vi "HFRR ADV v016 new software.vi"() -> ()   [LabVIEW 2025] (continued)
            n3512 = local read "S 49"() -> (w4506:string)
            n3513 = local read "S 52"() -> (w4503:string)
            n3514 = local read "as"() -> (w4488:string)
            n3515 = local read "bs"() -> (w4489:string)
            n3516 = local read "S 56"() -> (w4502:string)
            n3517 = local read "S 57"() -> (w4501:string)
            n3518 = local read "S 58"() -> (w4500:string)
            n3519 = local read "S 59"() -> (w4499:string)
            n3520 = property on="OPEN" class="Bool (strict)"("Boolean Text.Text"=w4503) -> ()  [unwired: 2 in, 2 out]
            n3521 = property on="OPEN 1" class="Bool (strict)"("Boolean Text.Text"=w4507) -> ()  [unwired: 2 in, 2 out]
            n3522 = property on="OPEN 2" class="Bool (strict)"("Boolean Text.Text"=w4506) -> ()  [unwired: 2 in, 2 out]
            n3523 = property on="OPEN 3" class="Bool (strict)"("Boolean Text.Text"=w4505) -> ()  [unwired: 2 in, 2 out]
            n3524 = property on="OPEN 4" class="Bool (strict)"("Boolean Text.Text"=w4504) -> ()  [unwired: 2 in, 2 out]
            n3525 = Concatenate Strings(w4489, "\r", w4488) -> ()  [unwired: 1 out]
            n3526 = local read "S 102"() -> (w4462:string)
            n3527 = property on="КОФ1" class="DigNum (strict)"("Caption.Text"=w4502) -> ()  [unwired: 2 in, 2 out]
            n3528 = local read "S 98"() -> (w4466:string)
            n3529 = local read "S 99"() -> (w4465:string)
            n3530 = local read "S 100"() -> (w4464:string)
            n3531 = local read "S 101"() -> (w4463:string)
            n3532 = property on="КОФ2" class="DigNum (strict)"("Caption.Text"=w4501) -> ()  [unwired: 2 in, 2 out]
            n3533 = property on="КОФ3" class="DigNum (strict)"("Caption.Text"=w4500) -> ()  [unwired: 2 in, 2 out]
            n3534 = property on="КОФ4" class="DigNum (strict)"("Caption.Text"=w4499) -> ()  [unwired: 2 in, 2 out]
            n3535 = local read "bs"() -> (w4487:string)
            n3536 = local read "as"() -> (w4486:string)
            n3537 = property on="CH-POWER +" class="DigNum (strict)"("Caption.Text"=w4466) -> ()  [unwired: 2 in, 2 out]
            n3538 = property on="CH-POWER -" class="DigNum (strict)"("Caption.Text"=w4465) -> ()  [unwired: 2 in, 2 out]
            n3539 = property on="CH-HEATER" class="DigNum (strict)"("Caption.Text"=w4464) -> ()  [unwired: 2 in, 2 out]
            n3540 = property on="CH-HUMIDITY DRY" class="DigNum (strict)"("Caption.Text"=w4463) -> ()  [unwired: 2 in, 2 out]
            n3541 = property on="CH-HUMIDITY WET" class="DigNum (strict)"("Caption.Text"=w4462) -> ()  [unwired: 2 in, 2 out]
            n3542 = local read "S 60"() -> (w4498:string)
            n3543 = local read "S 54"() -> (w4508:string)
            n3544 = Concatenate Strings(w4487, "\r", w4486) -> ()  [unwired: 1 out]
            n3545 = Concatenate Strings(w4508, w4498) -> ()  [unwired: 1 out]
            n3546 = local read "S 77"() -> (→"String 43":string)
            n3547 = local read "S 76"() -> (w4481:string)
            n3548 = local read "S 78"() -> (w4480:string)
            n3549 = local read "S 71"() -> (w4492:string)
            n3550 = local read "S 66"() -> (w4497:string)
            n3551 = local read "S 67"() -> (w4496:string)
            n3552 = local read "S 68"() -> (w4495:string)
            n3553 = local read "S 69"() -> (w4494:string)
            n3554 = local read "S 70"() -> (w4493:string)
            n3555 = property on="AIR TEMP" class="DigNum (strict)"("Caption.Text"=w4480) -> ()  [unwired: 2 in, 2 out]
            n3556 = property on="Set Strk" class="DigNum (strict)"("Caption.Text"=w4481) -> ()  [unwired: 2 in, 2 out]
            n3557 = property on="FRIC. FORCE :" class="DigNum (strict)"("Caption.Text"=w4497) -> ()  [unwired: 2 in, 2 out]
            n3558 = property on="TEMPERATURE :" class="DigNum (strict)"("Caption.Text"=w4496) -> ()  [unwired: 2 in, 2 out]
            n3559 = property on="SPEED OUT:" class="DigNum (strict)"("Caption.Text"=w4495) -> ()  [unwired: 2 in, 2 out]
            n3560 = property on="AIR TEMPERATURE :" class="DigNum (strict)"("Caption.Text"=w4494) -> ()  [unwired: 2 in, 2 out]
            n3561 = property on="HUMIDITY:" class="DigNum (strict)"("Caption.Text"=w4493) -> ()  [unwired: 2 in, 2 out]
            n3562 = property on="EDIT" class="Bool (strict)"("Boolean Text.Text"=w4492) -> ()  [unwired: 2 in, 2 out]
            n3563 = local read "S 79"() -> (w4479:string)
          }
          frame #2 {
          }
        }
        n3564 = local write "Lan flag"(10.0 ("Lan flag")) -> ()
      }
      frame Enabled {
      }
    }
    n3565 = Wait (ms)(milliseconds to wait=u32 2000) -> ()  [unwired: 1 out]
    n3566 = local read "Quit"() -> (w4282:bool)
  }
  n3567 = disable-structure shown="Disabled" {
    frame Disabled {
      n3568 = while {
        tunnel: [w4510] -> _
        i -> [w4510]
        stop <- w4509 continue-if-true
        n3569 = Wait (ms)(milliseconds to wait=u32 50) -> ()  [unwired: 1 out]
        n3570 = stacked-sequence {
          frame #0 {
            # "Controls Text color"
            # "Controls BG color"
            n3571 = property on="FILE" class="Str"("Text.Text Colors:Text Color"="SC  Text") -> ()  [unwired: 2 in, 2 out]
            n3572 = property on="Fuel Discription :" class="Str"("Text.Text Colors:Text Color"="SC  Text") -> ()  [unwired: 2 in, 2 out]
            n3573 = property on="tested by" class="Str"("Text.Text Colors:Text Color"="SC  Text") -> ()  [unwired: 2 in, 2 out]
            n3574 = property on="Remarks :" class="Str"("Text.Text Colors:Text Color"="SC  Text") -> ()  [unwired: 2 in, 2 out]
            n3575 = property class="DigNum (strict)"("Numeric Text.Text Colors:BG Color"="NC BG") -> ()  [unwired: 2 in, 2 out]
            n3576 = property class="DigNum (strict)"("Numeric Text.Text Colors:BG Color"="NC BG") -> ()  [unwired: 2 in, 2 out]
            n3577 = property class="DigNum (strict)"("Numeric Text.Text Colors:BG Color"="NC BG") -> ()  [unwired: 2 in, 2 out]
            n3578 = property class="DigNum (strict)"("Numeric Text.Text Colors:BG Color"="NC BG") -> ()  [unwired: 2 in, 2 out]
            n3579 = property class="DigNum (strict)"("Numeric Text.Text Colors:BG Color"="NC BG") -> ()  [unwired: 2 in, 2 out]
            n3580 = property class="DigNum (strict)"("Numeric Text.Text Colors:BG Color"="NC BG") -> ()  [unwired: 2 in, 2 out]
            n3581 = property class="DigNum (strict)"("Numeric Text.Text Colors:BG Color"="NC BG") -> ()  [unwired: 2 in, 2 out]
            n3582 = property class="DigNum (strict)"("Numeric Text.Text Colors:BG Color"="NC BG") -> ()  [unwired: 2 in, 2 out]
            n3583 = property class="DigNum (strict)"("Numeric Text.Text Colors:BG Color"="NC BG") -> ()  [unwired: 2 in, 2 out]
            n3584 = property class="DigNum (strict)"("Numeric Text.Text Colors:BG Color"="NC BG") -> ()  [unwired: 2 in, 2 out]
            n3585 = property class="DigNum (strict)"("Numeric Text.Text Colors:BG Color"="NC BG") -> ()  [unwired: 2 in, 2 out]
            n3586 = property class="DigNum (strict)"("Numeric Text.Text Colors:BG Color"="NC BG") -> ()  [unwired: 2 in, 2 out]
            n3587 = property on="FILE" class="Str"("Text.Text Colors:BG Color"="SC BG 3") -> ()  [unwired: 2 in, 2 out]
            n3588 = property on="Fuel Discription :" class="Str"("Text.Text Colors:BG Color"="SC BG 3") -> ()  [unwired: 2 in, 2 out]
            n3589 = property on="tested by" class="Str"("Text.Text Colors:BG Color"="SC BG 3") -> ()  [unwired: 2 in, 2 out]
            n3590 = property on="Remarks :" class="Str"("Text.Text Colors:BG Color"="SC BG 3") -> ()  [unwired: 2 in, 2 out]
            n3591 = property class="DigNum (strict)"("Numeric Text.Text Colors:Text Color"="NC Text") -> ()  [unwired: 2 in, 2 out]
            n3592 = property class="DigNum (strict)"("Numeric Text.Text Colors:Text Color"="NC Text") -> ()  [unwired: 2 in, 2 out]
            n3593 = property class="DigNum (strict)"("Numeric Text.Text Colors:Text Color"="NC Text") -> ()  [unwired: 2 in, 2 out]
            n3594 = property class="DigNum (strict)"("Numeric Text.Text Colors:Text Color"="NC Text") -> ()  [unwired: 2 in, 2 out]
            n3595 = property class="DigNum (strict)"("Numeric Text.Text Colors:Text Color"="NC Text") -> ()  [unwired: 2 in, 2 out]
            n3596 = property class="DigNum (strict)"("Numeric Text.Text Colors:Text Color"="NC Text") -> ()  [unwired: 2 in, 2 out]
            n3597 = property class="DigNum (strict)"("Numeric Text.Text Colors:Text Color"="NC Text") -> ()  [unwired: 2 in, 2 out]
            n3598 = property class="DigNum (strict)"("Numeric Text.Text Colors:Text Color"="NC Text") -> ()  [unwired: 2 in, 2 out]
            n3599 = property class="DigNum (strict)"("Numeric Text.Text Colors:Text Color"="NC Text") -> ()  [unwired: 2 in, 2 out]
            n3600 = property class="DigNum (strict)"("Numeric Text.Text Colors:Text Color"="NC Text") -> ()  [unwired: 2 in, 2 out]
            n3601 = property class="DigNum (strict)"("Numeric Text.Text Colors:Text Color"="NC Text") -> ()  [unwired: 2 in, 2 out]
            n3602 = property class="DigNum (strict)"("Numeric Text.Text Colors:Text Color"="NC Text") -> ()  [unwired: 2 in, 2 out]
            n3603 = property class="DigNum (strict)"("Numeric Text.Text Colors:Text Color"="NI Text  2") -> ()  [unwired: 2 in, 2 out]
            n3604 = property class="DigNum (strict)"("Numeric Text.Text Colors:Text Color"="NI Text  2") -> ()  [unwired: 2 in, 2 out]
            n3605 = property class="DigNum (strict)"("Numeric Text.Text Colors:Text Color"="NI Text  2") -> ()  [unwired: 2 in, 2 out]
            n3606 = property class="DigNum (strict)"("Numeric Text.Text Colors:Text Color"="NI Text  2") -> ()  [unwired: 2 in, 2 out]
            n3607 = property class="DigNum (strict)"("Numeric Text.Text Colors:Text Color"="NI Text  2") -> ()  [unwired: 2 in, 2 out]
            n3608 = property class="DigNum (strict)"("Numeric Text.Text Colors:Text Color"="NI Text  2") -> ()  [unwired: 2 in, 2 out]
            n3609 = property class="DigNum (strict)"("Numeric Text.Text Colors:Text Color"="NI Text  2") -> ()  [unwired: 2 in, 2 out]
            n3610 = property class="DigNum (strict)"("Numeric Text.Text Colors:Text Color"="NI Text  2") -> ()  [unwired: 2 in, 2 out]
            n3611 = property class="DigNum (strict)"("Numeric Text.Text Colors:Text Color"="NI Text  2") -> ()  [unwired: 2 in, 2 out]
            n3612 = property class="DigNum (strict)"("Numeric Text.Text Colors:Text Color"="NI Text  2") -> ()  [unwired: 2 in, 2 out]
            n3613 = property class="DigNum (strict)"("Numeric Text.Text Colors:Text Color"="NI Text  2") -> ()  [unwired: 2 in, 2 out]
            n3614 = property class="DigNum (strict)"("Numeric Text.Text Colors:Text Color"="NI Text  2") -> ()  [unwired: 2 in, 2 out]
            n3615 = property class="DigNum (strict)"("Numeric Text.Text Colors:Text Color"="NI Text  2") -> ()  [unwired: 2 in, 2 out]
            n3616 = property class="DigNum (strict)"("Numeric Text.Text Colors:Text Color"="NI Text  2") -> ()  [unwired: 2 in, 2 out]
            n3617 = property class="DigNum (strict)"("Numeric Text.Text Colors:Text Color"="NI Text  2") -> ()  [unwired: 2 in, 2 out]
            n3618 = property on="Coefficient Of Friction" class="XYGraph (strict)"("Plot Area:Colors:FG Color"="GFG  2", "Plot Area:Colors:BG Color"="GBG   2") -> ()  [unwired: 2 in, 2 out]
            n3619 = property on="Humidity ( %RH )" class="XYGraph (strict)"("Plot Area:Colors:FG Color"="GFG  2", "Plot Area:Colors:BG Color"="GBG   2") -> ()  [unwired: 2 in, 2 out]
            n3620 = property on="Air Temperature  ( °C )" class="XYGraph (strict)"("Plot Area:Colors:FG Color"="GFG  2", "Plot Area:Colors:BG Color"="GBG   2") -> ()  [unwired: 2 in, 2 out]
            n3621 = property on="Sample Temperature ( °C )" class="XYGraph (strict)"("Plot Area:Colors:FG Color"="GFG  2", "Plot Area:Colors:BG Color"="GBG   2") -> ()  [unwired: 2 in, 2 out]
            n3622 = property class="DigNum (strict)"("Numeric Text.Text Colors:BG Color"="NI BG 2") -> ()  [unwired: 2 in, 2 out]
            n3623 = property class="DigNum (strict)"("Numeric Text.Text Colors:BG Color"="NI BG 2") -> ()  [unwired: 2 in, 2 out]
            n3624 = property class="DigNum (strict)"("Numeric Text.Text Colors:BG Color"="NI BG 2") -> ()  [unwired: 2 in, 2 out]
            n3625 = property class="DigNum (strict)"("Numeric Text.Text Colors:BG Color"="NI BG 2") -> ()  [unwired: 2 in, 2 out]
            n3626 = property class="DigNum (strict)"("Numeric Text.Text Colors:BG Color"="NI BG 2") -> ()  [unwired: 2 in, 2 out]
            n3627 = property class="DigNum (strict)"("Numeric Text.Text Colors:BG Color"="NI BG 2") -> ()  [unwired: 2 in, 2 out]
            n3628 = property class="DigNum (strict)"("Numeric Text.Text Colors:BG Color"="NI BG 2") -> ()  [unwired: 2 in, 2 out]
            n3629 = property class="DigNum (strict)"("Numeric Text.Text Colors:BG Color"="NI BG 2") -> ()  [unwired: 2 in, 2 out]
            n3630 = property class="DigNum (strict)"("Numeric Text.Text Colors:BG Color"="NI BG 2") -> ()  [unwired: 2 in, 2 out]
            n3631 = property class="DigNum (strict)"("Numeric Text.Text Colors:BG Color"="NI BG 2") -> ()  [unwired: 2 in, 2 out]
            n3632 = property class="DigNum (strict)"("Numeric Text.Text Colors:BG Color"="NI BG 2") -> ()  [unwired: 2 in, 2 out]
            n3633 = property class="DigNum (strict)"("Numeric Text.Text Colors:BG Color"="NI BG 2") -> ()  [unwired: 2 in, 2 out]
            n3634 = property class="DigNum (strict)"("Numeric Text.Text Colors:BG Color"="NI BG 2") -> ()  [unwired: 2 in, 2 out]
            n3635 = property class="DigNum (strict)"("Numeric Text.Text Colors:BG Color"="NI BG 2") -> ()  [unwired: 2 in, 2 out]
            n3636 = property class="DigNum (strict)"("Numeric Text.Text Colors:BG Color"="NI BG 2") -> ()  [unwired: 2 in, 2 out]
            n3637 = property class="Bool"("Colors [4]"="Boolean BC T & BG") -> ()  [unwired: 2 in, 2 out]
            n3638 = property on="Save & Continue" class="Bool (strict)"("Colors [4]"="Boolean BC T & BG") -> ()  [unwired: 2 in, 2 out]
            n3639 = property on="Heater Button" class="Bool (strict)"("Colors [4]"="Boolean BC T & BG") -> ()  [unwired: 2 in, 2 out]
            n3640 = property class="Bool"("Colors [4]"="Boolean BC T & BG") -> ()  [unwired: 2 in, 2 out]
            n3641 = property on="Humidity" class="Bool (strict)"("Colors [4]"="Boolean BC T & BG") -> ()  [unwired: 2 in, 2 out]
            n3642 = property class="Bool (strict)"("Colors [4]"="Boolean BC T & BG") -> ()  [unwired: 2 in, 2 out]
            n3643 = property on="RUN" class="Bool (strict)"("Colors [4]"="Boolean BC T & BG") -> ()  [unwired: 2 in, 2 out]
            n3644 = property on="trip1 8" class="Bool (strict)"("Colors [4]"="Boolean BC T & BG") -> ()  [unwired: 2 in, 2 out]
            n3645 = property class="Bool"("Colors [4]"="Boolean BC T & BG") -> ()  [unwired: 2 in, 2 out]
            n3646 = property class="Bool (strict)"("Colors [4]"="Boolean BC T & BG") -> ()  [unwired: 2 in, 2 out]
            n3647 = property on="OPEN 1" class="Bool (strict)"("Colors [4]"="Boolean BC T & BG 2") -> ()  [unwired: 2 in, 2 out]
            n3648 = property on="OPEN 2" class="Bool (strict)"("Colors [4]"="Boolean BC T & BG 2") -> ()  [unwired: 2 in, 2 out]
            n3649 = property on="OPEN 3" class="Bool (strict)"("Colors [4]"="Boolean BC T & BG 2") -> ()  [unwired: 2 in, 2 out]
            n3650 = property on="OPEN 4" class="Bool (strict)"("Colors [4]"="Boolean BC T & BG 2") -> ()  [unwired: 2 in, 2 out]
            n3651 = property on="OPEN" class="Bool (strict)"("Colors [4]"="Boolean BC T & BG 2") -> ()  [unwired: 2 in, 2 out]
            n3652 = property on="rstv2" class="Bool"("Colors [4]"="Boolean BC T & BG 2") -> ()  [unwired: 2 in, 2 out]
            n3653 = property on="RST CP" class="Bool"("Colors [4]"="Boolean BC T & BG 2") -> ()  [unwired: 2 in, 2 out]
            n3654 = property on="RSTV1 3" class="Bool"("Colors [4]"="Boolean BC T & BG 2") -> ()  [unwired: 2 in, 2 out]
            n3655 = property on="RSTV1 2" class="Bool"("Colors [4]"="Boolean BC T & BG 2") -> ()  [unwired: 2 in, 2 out]
          }
          frame #1 {
          }
        }
        n3656 = local read "Quit"() -> (w4509:bool)
      }
    }
    frame Enabled {
    }
  }
  n3657 = while {
    shift-right: [w4527] -> _
    shift-left: _ -> [w4528]
    shift-right: [w4525] -> _
    shift-left: T19 {"Read Heave and Surge"="", "Bytes at Heave Port"=0.0, "Heave and Surge COM Port:"="COM9", "Com Port 2"="COM7", "Residual Due"="", "Heave COM Status 2"=TRUE, "Heave COM Status"=TRUE, "Port 2"=TRUE, "Sway PPR"=6400.0, "Surge PPR"=6400.0, "Heave PPR"=6400.0, "Sway Pitch"=2.0, "Surge Pitch"=3.0, "Heave Pitch"=4.0, "Sway Pulses/mm"=320.0, "Surge Pulses/mm"=1600.0, "Heave Pulses/mm"=1600.0, "inner loop"=0.0, "Read Heave and Surge 2"="", "String 36"="", "Write S"=FALSE, "WriteCC1"=[""], "Heave COM Loop"=0, "LastCom"="", "EXIT"=FALSE, "Error Heave"={"status"=TRUE, "code"=-1073807343, "source"=""}} -> [w4524]
    shift-right: [w4522] -> _
    shift-left: enum16{"init", "MAIN", "Panel Close"}."init" -> [w4523]
    stop <- w4526 stop-if-true
    n3658 = case shown="\"MAIN\"" w4523 {
      tunnel: w4528 -> [w4542 w4557 w4618 w4620]
      tunnel: [w4536 w4566 w4618 w4620] -> w4527
      tunnel: [_ _ TRUE _] -> w4526
      tunnel: [w4532 w4563 w4616 w4619] -> w4525
      tunnel: w4524 -> [w4539 w4556 w4616 w4619]
      tunnel: [enum16{"init", "MAIN", "Panel Close"}."MAIN" w4550 _ _] -> w4522
      frame "init" {
        n3659 = Bundle By Name(cluster=w4539, "Heave and Surge COM Port:"="C3 :") -> (w4538:T19)
        n3660 = call "Instrument fgv.vi"("Enum"=T31."INIT", "error in (no error) 2"=w4542, "INPUT"=w4538) -> ("error"=w4540:errorcluster, "output"=w4535:T19)  [unwired: 6 in, 1 out]
        n3661 = case shown="Error" w4540 {
          selector: w4540 -> [w4544 _]
          tunnel: [w4544 w4548] -> w4536
          tunnel: w4535 -> [w4543 w4546]
          tunnel: [w4543 w4545] -> w4533
          frame No Error {
          }
          frame Error {
            n3662 = call "Instrument fgv.vi"("Enum"=T31."ERROR INIT", "INPUT"=w4546) -> ("error"=w4549:errorcluster, "output"=w4545:T19)  [unwired: 7 in, 1 out]
            n3663 = call <vilib>:"Clear Errors.vi"("error in (no error)"=w4549) -> ("error out"=w4548:errorcluster)  [unwired: 5 in, 1 out]
          }
        }
        n3664 = local read "LastCom"() -> (w4531:string)
        n3665 = Unbundle By Name(w4533) -> ("Heave COM Status 2"=→"COM Status" →"Instrument Status":bool, "Error Heave"=→"Error":errorcluster)  [unwired: 1 out]
        n3666 = Bundle By Name(cluster=w4533, "LastCom"=w4531) -> (w4532:T19)
      }
      frame "MAIN" {
        n3667 = Unbundle By Name(w4556) -> ("Com Port 2"=w4568:refnum<visa-resource-name>)
        n3668 = local write "Com Port 4"(w4568) -> ()
        n3669 = local read "C3 :"() -> (w4554:refnum<visa-resource-name>)
        n3670 = Bundle By Name(cluster=w4556, "Heave and Surge COM Port:"=w4554) -> (w4555:T19)
        n3671 = Equal?(x=w4568, y=w4554) -> (x = y?=w4567:bool)
        n3672 = case shown="True" w4567 {
          tunnel: [w4572 w4589] -> w4566
          tunnel: w4557 -> [w4573 w4595]
          tunnel: w4555 -> [w4571 w4593]
          tunnel: [w4570 w4588] -> w4563
          frame False {
            n3673 = call <vilib>:"Clear Errors.vi"("error in (no error)"=w4573) -> ("error out"=w4569:errorcluster)  [unwired: 5 in, 1 out]
            n3674 = call "Instrument fgv.vi"("Enum"=T31."ERROR INIT", "error in (no error) 2"=w4569, "INPUT"=w4571) -> ("error"=w4575:errorcluster, "output"=w4570:T19)  [unwired: 6 in, 1 out]
            n3675 = call <vilib>:"Clear Errors.vi"("error in (no error)"=w4575) -> ("error out"=w4572:errorcluster)  [unwired: 5 in, 1 out]
          }
          frame True {
            n3676 = call "Instrument fgv.vi"("Enum"=T31."READ", "error in (no error) 2"=w4595, "INPUT"=w4593) -> ("error"=w4594:errorcluster, "output"=w4585:T19)  [unwired: 6 in, 1 out]
            n3677 = Bundle By Name(cluster=w4585, "String 36"="String 11") -> (w4584:T19)
            n3678 = case shown="True" "Write S" {
              selector: "Write S" -> [_ w4615]
              tunnel: w4594 -> [w4608 w4614]
              tunnel: [w4608 w4613] -> w4581
              tunnel: w4584 -> [w4607 w4610]
              tunnel: [w4607 w4609] -> w4580
              frame False {
              }
              frame True {
                n3679 = Not(x=w4615) -> (.not. x?=w4611:bool)
                n3680 = local write "Write S"(w4611) -> ()
                n3681 = call "Instrument fgv.vi"("Enum"=T31."MANUAL WRITE", "error in (no error) 2"=w4614, "INPUT"=w4610) -> ("error"=w4613:errorcluster, "output"=w4609:T19)  [unwired: 6 in, 1 out]
              }
            }
            n3682 = Array Size(array="WriteHumidity") -> (size(s)=w4578:i32)
            n3683 = Greater Than 0?(x=w4578) -> (x > 0?=w4576:bool)
            n3684 = call "Instrument fgv.vi"("Enum"=T31."WRITE", "error in (no error) 2"=w4581, "WriteCC1"="WriteHumidity", "INPUT"=w4580) -> ("error"=w4591:errorcluster, "WriteCC1 2"=w4579:string[], "output"=w4590:T19)  [unwired: 5 in]
            n3685 = case shown="True" w4576 {
              tunnel: w4579 -> [_ w4597]
              frame False {
              }
              frame True {
                n3686 = local write "WriteHumidity"(w4597) -> ()
              }
            }
            n3687 = case shown="Error" w4591 {
              selector: w4591 -> [w4598 w4601]
              tunnel: w4590 -> [w4599 w4606]
              tunnel: [w4599 w4605] -> w4588
              tunnel: [w4598 w4603] -> w4589
              frame No Error {
              }
              frame Error {
                n3688 = call <vilib>:"Clear Errors.vi"("error in (no error)"=w4601) -> ("error out"=w4600:errorcluster)  [unwired: 5 in, 1 out]
                n3689 = call "Instrument fgv.vi"("Enum"=T31."ERROR INIT", "error in (no error) 2"=w4600, "INPUT"=w4606) -> ("error"=w4604:errorcluster, "output"=w4605:T19)  [unwired: 6 in, 1 out]
                n3690 = call <vilib>:"Clear Errors.vi"("error in (no error)"=w4604) -> ("error out"=w4603:errorcluster)  [unwired: 5 in, 1 out]
              }
            }
            n3691 = Unbundle By Name(w4588) -> ("LastCom"=→"LastCom":string, "Read Heave and Surge"=→"Read Humidity":string)
          }
        }
        n3692 = Unbundle By Name(w4563) -> ("Heave COM Status 2"=w4565:bool, "Heave COM Status"=w4564:bool, "Error Heave"=w4561:errorcluster, "Bytes at Heave Port"=→"Bytes at Humidity Port":dbl)
        n3693 = Unbundle By Name(w4561) -> ("status"=→"Humidity Port":bool)
        n3694 = Not(x=w4564) -> (.not. x?=w4558:bool)
        n3695 = local write "Error"(w4561) -> ()
        n3696 = Not(x=w4565) -> (.not. x?=w4559:bool)
        n3697 = local write "Instrument Status"(w4558) -> ()
        n3698 = local write "COM Status"(w4559) -> ()
        n3699 = local read "Quit"() -> (w4551:bool)
        n3700 = Select(t=enum16{"init", "MAIN", "Panel Close"}."Panel Close", s=w4551, f=enum16{"init", "MAIN", "Panel Close"}."MAIN") -> (s? t:f=w4550:enum16{"init", "MAIN", "Panel Close"})
      }
      frame "Panel Close" {
      }
      frame Default {
      }
    }
  }
  n3701 = while {
    stop <- w4646 stop-if-true
    n3702 = local read "Read Humidity"() -> (w4627:string)
    n3703 = call <vilib>:"High Resolution Polling Wait.vi"("seconds to wait"=0.1) -> ()  [unwired: 10 in, 1 out]
    n3704 = Spreadsheet String To Array(delimiter (Tab)=",", format string="", spreadsheet string=w4627, array type (2D Dbl)=string[] []) -> (array=w4641:string[])
    n3705 = for {
      tunnel: w4641 -> [w4651] mode=indexing
      tunnel: string[] ["STATE;", "SET;", "RH;", "T;", "AMB_RH;", "AMB_T;", "PUMP;", "FAN_IN;", "FAN_OUT;", "DEHUM;", "CURRENT;", "STALL;"] -> [w4650] mode=indexing
      tunnel: [w4649] -> w4640 mode=indexing
      n3706 = Match Pattern(string=w4651, regular expression=w4650) -> (after substring=w4649:string)  [unwired: 1 in, 3 out]
    }
    n3707 = Index Array(array=w4640) -> (element #1=→"STATE :":string, element #2=→"SET :":string, element #3=w4629:string, element #4=→"T :":string, element #5=w4626:string, element #6=→"AMB_T :":string, element #7=→"PUMP :":string, element #8=→"FAN_IN :":string, element #9=→"FAN_OUT :":string, element #10=→"DEHUM :":string, element #11=→"CURRENT :":string, element #12=→"STALL :":string)  [unwired: 12 in]
    "RH :" <- w4629
    "AMB_RH :" <- w4626
    n3708 = Fract/Exp String To Number(string=w4629) -> (number=w4621:dbl)  [unwired: 3 in, 1 out]
    n3709 = Fract/Exp String To Number(string=w4626) -> (number=w4625:dbl)  [unwired: 3 in, 1 out]
    n3710 = local write "Ambient Humidity :"(w4625) -> ()
    n3711 = Equal?(x=w4621, y=0.0) -> (x = y?=w4623:bool)
    n3712 = case shown="True" w4623 {
      tunnel: [w4647 w4648] -> w4622
      tunnel: w4621 -> [w4647 _]
      frame False {
        (unwired) 0.0
        "Humidity temp" <- w4647
      }
      frame True {
        n3713 = local read "Humidity temp"() -> (w4648:dbl)
      }
    }
    "RH Numeric:" <- w4622
    n3714 = local read "Quit"() -> (w4646:bool)
  }
  n3715 = disable-structure shown="Disabled" {
    frame Disabled {
      n3716 = while {
        tunnel: [w4885] -> _
        i -> [w4885]
        stop <- w4882 stop-if-true
        n3717 = local read "powstat"() -> (w4883:bool)
        n3718 = case shown="True" w4883 {
          frame False {
          }
          frame True {
            n3719 = local read "RUN"() -> (w4886:bool)
            n3720 = case shown="True" w4886 {
              frame False {
                w4916 = 65.0 ("y")
                n3721 = local read "Set Hz"() -> (w4944:dbl)
                n3722 = local read "NORMAL LOAD"() -> (w4945:dbl)
                n3723 = Multiply(x=w4944, y=60.0) -> (x*y=w4951:dbl)
                n3724 = Multiply(x=1.2 ("y"), y=0.949) -> (x*y=w4920:dbl)
                n3725 = Multiply(x=1.2 ("y"), y=0.8166) -> (x*y=w4924:dbl)
                n3726 = Multiply(x=1.2 ("y"), y=0.851) -> (x*y=w4919:dbl)
                n3727 = local read "FF 2"() -> (w4943:dbl)
                n3728 = Absolute Value(x=w4951) -> (abs(x)=w4949:dbl)
                n3729 = case shown="13.." w4943 {
                  tunnel: [1 2 3] -> w4941
                  frame 0..10, Default {
                    # "Normal"
                  }
                  frame 11, 12 {
                  }
                  frame 13.. {
                  }
                }
                "FF STATE" <- w4941
                n3730 = local read "TEMP"() -> (w4904:dbl)
                n3731 = local read item#-1() -> (w4918)
                n3732 = Less?(x=w4918, y=w4924) -> (x < y?=w4921:bool)
                n3733 = In Range and Coerce(upper limit=w4920, x=w4918, lower limit=w4919) -> (In Range?=w4922:bool)  [unwired: 1 out]
                n3734 = case shown="3601.." w4949 {
                  tunnel: [1 2 3] -> w4947
                  frame 0..3000, Default {
                    # "Normal"
                  }
                  frame 3001..3600 {
                  }
                  frame 3601.. {
                  }
                }
                n3735 = case shown="11.." w4945 {
                  tunnel: [1 3] -> w4946
                  frame 1..10, Default {
                  }
                  frame 11.. {
                  }
                }
                "NL STATE" <- w4946
                n3736 = Multiply(x=1.2 ("y"), y=0.95) -> (x*y=w4934:dbl)
                n3737 = Multiply(x=w4916, y=0.954) -> (x*y=w4908:dbl)
                n3738 = Or(x=w4921, y=w4922) -> (x .or. y?=w4923:bool)
                n3739 = Greater Or Equal?(x=w4918, y=w4934) -> (x >= y?=w4931:bool)
                n3740 = Multiply(x=w4916, y=0.99) -> (x*y=w4905:dbl)
                n3741 = Greater Or Equal?(x=w4904, y=w4905) -> (x >= y?=w4910:bool)
                n3742 = Greater Or Equal?(x=w4904, y=w4908) -> (x >= y?=w4907:bool)
                n3743 = case shown="0, 1, Default" w4918 {
                  tunnel: [1 3] -> w4935
                  frame 0, 1, Default {
                  }
                  frame 2.. {
                  }
                }
                n3744 = case shown="True" w4931 {
                  tunnel: [1 3] -> w4936
                  frame False {
                  }
                  frame True {
                  }
                }
                n3745 = case shown="True" w4923 {
                  tunnel: [1 2] -> w4937
                  frame False {
                  }
                  frame True {
                  }
                }
                n3746 = case shown="..0" w4904 {
                  tunnel: [2 3 3 1] -> w4911
                  frame 61, 62 {
                  }
                  frame 63.. {
                  }
                  frame ..0 {
                  }
                  frame 10..60, Default {
                  }
                }
                n3747 = case shown="True" w4910 {
                  tunnel: [1 3] -> w4912
                  frame False {
                  }
                  frame True {
                  }
                }
                n3748 = Number To Decimal String(number=w4947) -> (decimal integer string=w4948:string)  [unwired: 1 in]
                n3749 = case shown="True" w4907 {
                  tunnel: [1 2] -> w4913
                  frame False {
                  }
                  frame True {
                  }
                }
                n3750 = Number To Decimal String(number=1) -> (decimal integer string=→"Air temp":string)  [unwired: 1 in]
                n3751 = Number To Decimal String(number=w4941) -> (decimal integer string=→"ff_st":string)  [unwired: 1 in]
                n3752 = local write "sp_st"(w4948) -> ()
                n3753 = Number To Decimal String(number=w4946) -> (decimal integer string=→"nl_st":string)  [unwired: 1 in]
                n3754 = Build Array(w4911, w4912, w4913) -> (w4914:i32[])
                n3755 = Build Array(w4935, w4936, w4937) -> (w4938:i32[])
                n3756 = Array Max & Min(array=w4914) -> (max value=w4915:i32)  [unwired: 3 out]
                n3757 = Array Max & Min(array=w4938) -> (max value=w4939:i32)  [unwired: 3 out]
                n3758 = Number To Decimal String(number=w4915) -> (decimal integer string=w4903:string)  [unwired: 1 in]
                n3759 = Number To Decimal String(number=w4939) -> (decimal integer string=→"Stroke Ln 2":string)  [unwired: 1 in]
                n3760 = local write "temp_st"(w4903) -> ()
              }
              frame True {
                w5001 = 65.0 ("y")
                # "Healthy -1\nWarning -2\nError -3"
                n3761 = local read "TEMP"() -> (w5012:dbl)
                n3762 = local read "NORMAL LOAD"() -> (w5016:dbl)
                n3763 = local read "Set Hz"() -> (w5014:dbl)
                n3764 = Multiply(x=1.2 ("y"), y=0.949) -> (x*y=w4996:dbl)
                n3765 = Multiply(x=1.2 ("y"), y=0.8166) -> (x*y=w4992:dbl)
                n3766 = Multiply(x=1.2 ("y"), y=0.851) -> (x*y=w4997:dbl)
                n3767 = Multiply(x=w5001, y=0.954) -> (x*y=w5008:dbl)
                n3768 = Multiply(x=w5001, y=0.99) -> (x*y=w5011:dbl)
                n3769 = Greater Or Equal?(x=w5012, y=w5011) -> (x >= y?=w5006:bool)
                n3770 = Multiply(x=w5014, y=60.0) -> (x*y=w5020:dbl)
                n3771 = Greater Or Equal?(x=w5012, y=w5008) -> (x >= y?=w5009:bool)
                n3772 = local read "FF 2"() -> (w5015:dbl)
                n3773 = local read item#-1() -> (w4998)
                n3774 = Less?(x=w4998, y=w4992) -> (x < y?=w4995:bool)
                n3775 = In Range and Coerce(upper limit=w4996, x=w4998, lower limit=w4997) -> (In Range?=w4994:bool)  [unwired: 1 out]
                n3776 = Absolute Value(x=w5020) -> (abs(x)=w5018:dbl)
                n3777 = case shown="63.." w5012 {
                  tunnel: [2 3 3 1] -> w5005
                  frame 61, 62 {
                  }
                  frame 63.. {
                  }
                  frame ..0 {
                  }
                  frame 10..60, Default {
                  }
                }
                n3778 = case shown="True" w5006 {
                  tunnel: [1 3] -> w5004
                  frame False {
                  }
                  frame True {
                  }
                }
                n3779 = case shown="True" w5009 {
                  tunnel: [1 2] -> w5003
                  frame False {
                  }
                  frame True {
                  }
                }
                n3780 = Multiply(x=1.2 ("y"), y=0.95) -> (x*y=w4982:dbl)
                n3781 = case shown="1..10, Default" w5016 {
                  tunnel: [1 3] -> w5023
                  frame 1..10, Default {
                  }
                  frame 11.. {
                  }
                }
                n3782 = case shown="0..10, Default" w5015 {
                  tunnel: [1 2 3] -> w5022
                  frame 0..10, Default {
                  }
                  frame 11, 12 {
                  }
                  frame 13.. {
                  }
                }
                n3783 = case shown="3601.." w5018 {
                  tunnel: [1 2 3] -> w5017
                  frame 0..3000, Default {
                    # "Normal"
                  }
                  frame 3001..3600 {
                  }
                  frame 3601.. {
                  }
                }
                n3784 = Or(x=w4995, y=w4994) -> (x .or. y?=w4993:bool)
                n3785 = Greater Or Equal?(x=w4998, y=w4982) -> (x >= y?=w4985:bool)
                n3786 = case shown="0, 1, Default" w4998 {
                  tunnel: [1 3] -> w4981
                  frame 0, 1, Default {
                  }
                  frame 2.. {
                  }
                }
                n3787 = case shown="True" w4985 {
                  tunnel: [1 3] -> w4980
                  frame False {
                  }
                  frame True {
                  }
                }
                n3788 = case shown="True" w4993 {
                  tunnel: [1 2] -> w4979
                  frame False {
                  }
                  frame True {
                  }
                }
                n3789 = Build Array(w5005, w5004, w5003) -> (w5002:i32[])
                n3790 = Number To Decimal String(number=w5017) -> (decimal integer string=→"sp_st":string)  [unwired: 1 in]
                n3791 = Array Max & Min(array=w5002) -> (max value=w4999:i32)  [unwired: 3 out]
                "TEMP STATE" <- w4999
                n3792 = Number To Decimal String(number=w5023) -> (decimal integer string=w5026:string)  [unwired: 1 in]
                n3793 = Number To Decimal String(number=w5022) -> (decimal integer string=w5024:string)  [unwired: 1 in]
                n3794 = Number To Decimal String(number=w4999) -> (decimal integer string=→"temp_st":string)  [unwired: 1 in]
                n3795 = Build Array(w4981, w4980, w4979) -> (w4978:i32[])
                n3796 = local write "nl_st"(w5026) -> ()
                n3797 = local write "ff_st"(w5024) -> ()
                n3798 = Number To Decimal String(number=1) -> (decimal integer string=w5021:string)  [unwired: 1 in]
                n3799 = Array Max & Min(array=w4978) -> (max value=w4977:i32)  [unwired: 3 out]
                n3800 = local write "Air temp"(w5021) -> ()
                n3801 = Number To Decimal String(number=w4977) -> (decimal integer string=w4976:string)  [unwired: 1 in]
                n3802 = local write "Stroke Ln 2"(w4976) -> ()
              }
            }
            n3803 = local read "Stroke Ln 2"() -> (w4888:string)
            n3804 = local read "nl_st"() -> (w4894:string)
            n3805 = local read "ff_st"() -> (w4891:string)
            n3806 = local read "sp_st"() -> (w4892:string)
            n3807 = local read "temp_st"() -> (w4893:string)
            n3808 = local read "Air temp"() -> (w4887:string)
            n3809 = Replace Array Subset(array="in", new element #1=w4894, index #1=1 ("index"), new element #2=w4891, index #2=2 ("index"), new element #3=w4893, index #3=3 ("index"), new element #4=w4892, index #4=4 ("index"), new element #5=w4888, index #5=5 ("index"), new element #6=w4887, index #6=6 ("index"), new element #7="Sensor State" ("new element/subarray"), index #7=0 ("index")) -> (→"out":string[])
          }
        }
        n3810 = Wait (ms)(milliseconds to wait=u32 10) -> ()  [unwired: 1 out]
        n3811 = local read "Quit"() -> (w4882:bool)
      }
      n3812 = while {
        stop <- w4857 stop-if-true
        n3813 = local read "run replace"() -> (w4859:bool)
        n3814 = Wait (ms)(milliseconds to wait=u32 100) -> ()  [unwired: 1 out]
        n3815 = Equal?(x="FLAG 2", y=0.0) -> (x = y?=w4860:bool)
        n3816 = case shown="True" w4860 {
          frame False {
          }
          frame True {
            n3817 = local write "FLAG 2"(100.0 ("FLAG 2")) -> ()
            n3818 = call <vilib>:"Read Characters From File.vi"("file path (dialog if empty)"=path "C:/LAB-IQ-NXT/WO 2449 TT.sig", "convert eol? (no:F)"=FALSE ("append to file? (new file:F)")) -> ("character string"=w4863:string)  [unwired: 4 in, 3 out]
            n3819 = call <vilib>:"Read Characters From File.vi"("file path (dialog if empty)"=path "C:/LAB-IQ-NXT/WO 2449 TRH.sig", "convert eol? (no:F)"=FALSE ("append to file? (new file:F)")) -> ("character string"=w4864:string)  [unwired: 4 in, 3 out]
            n3820 = Decimal String To Number(string=w4863) -> (number=w4865:i32)  [unwired: 2 in, 1 out]
            n3821 = local write "Total No. of Tests"(w4865) -> ()
            n3822 = Decimal String To Number(string=w4864) -> (number=w4868:i32)  [unwired: 2 in, 1 out]
            n3823 = local write "SEN.RUN HRS"(w4868) -> ()
          }
        }
        n3824 = case shown="True" w4859 {
          frame False {
          }
          frame True {
            n3825 = Equal?(x="FLAG 4", y=0.0) -> (x = y?=w4872:bool)
            n3826 = case shown="False" w4872 {
              frame False {
                n3827 = Get Date/Time In Seconds() -> (seconds since 1Jan1904=w4878:timestamp)
                n3828 = local read "START 3"() -> (w4876:dbl)
                n3829 = To Double Precision Float(number=w4878) -> (double precision float=w4877:dbl)
                n3830 = Subtract(x=w4877, y=w4876) -> (x-y=→"SENSOR TIME":dbl)
              }
              frame True {
                n3831 = Get Date/Time In Seconds() -> (seconds since 1Jan1904=w4880:timestamp)
                n3832 = local write "FLAG 4"(100.0 ("FLAG")) -> ()
                n3833 = To Double Precision Float(number=w4880) -> (double precision float=→"START 3":dbl)
              }
            }
          }
        }
        n3834 = local read "Quit"() -> (w4857:bool)
      }
      n3835 = while {
        shift-right: [w4657] -> _
        shift-left: _ -> [w4658]
        tunnel: [w4653] -> _
        i -> [w4653]
        stop <- w4652 stop-if-true
        n3836 = Wait (ms)(milliseconds to wait=u32 50 ("Refresh Rate (ms)")) -> ()  [unwired: 1 out]
        n3837 = local read "Json End Flg"() -> (w4654:bool)
        n3838 = Not(x="Upld AR 2") -> ()  [unwired: 1 out]
        n3839 = local read "Upld AR 2"() -> (w4655:bool)
        n3840 = call "Elapsed Time9"("Time Target (s)"="Sen.Upload Rate (s)", "Reset"=FALSE, "Auto Reset"=TRUE) -> ("Time has Elapsed"=w4664:bool)  [unwired: 9 in, 7 out]
        n3841 = Or(x=w4664, y=w4654) -> (x .or. y?=w4660:bool)
        n3842 = case shown="True" w4660 {
          frame False {
          }
          frame True {
            w4756 = "\"SensorName\":\"" ("string")
            w4726 = " \"},{"
            w4751 = "\",\"SensorState\":\""
            w4753 = "\",\"SensorModelNumber\":\"" ("string")
            w4752 = "\",\"SensorRuntimeHours\":\"" ("string")
            n3843 = local read "model num"() -> (w4750:string[])
            n3844 = local read "Sensor name"() -> (w4769:string[])
            n3845 = local read "run"() -> (w4740:string[])
            n3846 = local read "SENSOR TIME"() -> (w4696:dbl)
            n3847 = local read "out"() -> (w4689:string[])
            n3848 = local read "Total No. of Tests"() -> (w4694:dbl)
            n3849 = Select(t=60.0, s="Run test 3", f=3600.0) -> (s? t:f=w4704:dbl)
            n3850 = Index Array(array=w4750, index #1=1 ("index")) -> (element #1=w4749:string, element #2=w4748:string, element #3=w4747:string, element #4=w4746:string, element #5=w4745:string, element #6=w4744:string)  [unwired: 5 in]
            n3851 = Index Array(array=w4740, index #1=1 ("index")) -> (element #1=w4739:string, element #2=w4738:string, element #3=w4737:string, element #4=w4736:string, element #5=w4735:string, element #6=w4734:string)  [unwired: 5 in]
            n3852 = Index Array(array=w4769, index #1=1 ("index")) -> (element #1=w4768:string, element #2=w4767:string, element #3=w4766:string, element #4=w4765:string, element #5=w4755:string, element #6=w4754:string)  [unwired: 5 in]
            n3853 = Index Array(array=w4689, index #1=1 ("index")) -> (element #1=w4721:string, element #2=w4720:string, element #3=w4719:string, element #4=w4718:string, element #5=w4717:string, element #6=w4716:string)  [unwired: 5 in]
            n3854 = local read "SEN.RUN HRS"() -> (w4692:dbl)
            n3855 = Divide(x=w4696, y=w4704) -> (x/y=w4703:dbl)
            n3856 = Increment(x=w4703) -> (x+1=w4699:dbl)
            n3857 = Number To Decimal String(number=w4699) -> (decimal integer string=→"run hrs":string)  [unwired: 1 in]
            n3858 = Divide(x=w4692, y=3600.0 ("f")) -> (x/y=w4687:dbl)
            n3859 = Round To Nearest(number=w4687) -> (nearest integer value=w4685:dbl)
            n3860 = Number To Decimal String(number=w4685) -> (decimal integer string=w4686:string)  [unwired: 1 in]
            n3861 = Number To Decimal String(number=w4694) -> (decimal integer string=w4695:string)  [unwired: 1 in]
            n3862 = local read "Model No"() -> (w4700:string)
            n3863 = local read "UUID"() -> (w4795:string)
            n3864 = local read "Serial No"() -> (w4799:string)
            n3865 = local read "Secret Key"() -> (w4800:string)
            n3866 = Concatenate Strings("\",\"MachineSerialNumber\":\"" ("string"), w4799) -> (w4803:string)
            n3867 = Concatenate Strings("\",\"ModelNumber\":\"" ("string"), w4700) -> (w4701:string)
            n3868 = Concatenate Strings("\",\"MachineRuntimeHours\":\"" ("string"), w4686) -> (w4804:string)
            n3869 = Concatenate Strings("\",\"MachineRuntimeCycles\":\"", w4695) -> (w4797:string)
            n3870 = Concatenate Strings(w4753, w4749) -> (w4783:string)
            n3871 = Concatenate Strings(w4752, w4739) -> (w4784:string)
            n3872 = Concatenate Strings(w4751, w4721) -> (w4782:string)
            n3873 = Concatenate Strings(w4803, w4701, w4804, w4797) -> (w4806:string)
            n3874 = Concatenate Strings(w4753, w4748) -> (w4780:string)
            n3875 = Concatenate Strings(w4752, w4738) -> (w4779:string)
            n3876 = Concatenate Strings(w4751, w4720) -> (w4781:string)
            n3877 = Concatenate Strings(w4753, w4747) -> (w4775:string)
            n3878 = Concatenate Strings(w4752, w4737) -> (w4776:string)
            n3879 = Concatenate Strings(w4751, w4719) -> (w4774:string)
            n3880 = Concatenate Strings(w4753, w4746) -> (w4772:string)
            n3881 = Concatenate Strings(w4752, w4736) -> (w4771:string)
            n3882 = Concatenate Strings(w4751, w4718) -> (w4773:string)
            n3883 = Concatenate Strings(w4783, w4784, w4782) -> (w4785:string)
            n3884 = Concatenate Strings(w4753, w4745) -> (w4762:string)
            n3885 = Concatenate Strings(w4752, w4735) -> (w4763:string)
            n3886 = Concatenate Strings(w4753, w4744) -> (w4759:string)
            n3887 = Concatenate Strings(w4752, w4734) -> (w4758:string)
            n3888 = Concatenate Strings(w4751, w4717) -> (w4761:string)
            n3889 = Concatenate Strings(w4751, w4716) -> (w4760:string)
            n3890 = Concatenate Strings("{\"SecretKey\":\"", w4800, w4806, "\",\"UUID\" : \"", w4795, "\",\"SensorInformation\":", "[{" ("string")) -> (w4733:string)
            n3891 = Concatenate Strings(w4780, w4779, w4781) -> (w4778:string)
            n3892 = Concatenate Strings(w4775, w4776, w4774) -> (w4777:string)
            n3893 = Concatenate Strings(w4772, w4771, w4773) -> (w4770:string)
            n3894 = Concatenate Strings(w4762, w4763, w4761) -> (w4764:string)
            n3895 = Concatenate Strings(w4759, w4758, w4760) -> (w4757:string)
            n3896 = Concatenate Strings(w4756, w4768, w4785, w4726) -> (w4732:string)
            n3897 = Concatenate Strings(w4756, w4767, w4778, w4726) -> (w4731:string)
            n3898 = Concatenate Strings(w4756, w4766, w4777, w4726) -> (w4730:string)
            n3899 = Concatenate Strings(w4756, w4765, w4770, w4726) -> (w4729:string)
            n3900 = Concatenate Strings(w4756, w4755, w4764, w4726) -> (w4728:string)
            n3901 = Concatenate Strings(w4756, w4754, w4757, "\"}" ("string")) -> (w4727:string)
            n3902 = Concatenate Strings(w4733, w4732, w4731, w4730, w4729, w4728, w4727, "]}" ("string")) -> (w4724:string)
            n3903 = local read "SEN.RUN HRS"() -> (w4691:dbl)
            n3904 = disable-structure shown="Disabled" {
              frame Disabled {
                n3905 = local read "state"() -> (w4810:string[])
                n3906 = Delete From Array(array=w4810, index=0) -> (array with subset deleted=w4808:string[])  [unwired: 1 in, 1 out]
                n3907 = for {
                  N: 6 -> [_]
                  tunnel: w4808 -> [w4821] mode=indexing
                  tunnel: [w4820] -> w4807 mode=indexing
                  n3908 = Equal?(x=w4821, y="Warning") -> (x = y?=w4817:bool)
                  n3909 = Equal?(x=w4821, y="Healthy") -> (x = y?=w4814:bool)
                  n3910 = Select(t="2" ("y"), s=w4817, f="3" ("y")) -> (s? t:f=w4812:string)
                  n3911 = Select(t="1" ("y"), s=w4814, f=w4812) -> (s? t:f=w4820:string)
                }
                "state1" <- w4807
              }
              frame Enabled {
              }
            }
            n3912 = stacked-sequence {
              tunnel: w4724 -> [w4832 _ _]
              tunnel: [_ _ w4848] -> _
              frame #0 {
                (unwired) FALSE ("convert eol (F)")
                w4834 = enum16{"start", "end", "current"}."start" ("pos mode (0:2)")
                n3913 = local read "Path"() -> (w4828:path)
                n3914 = Path To String(path=w4828) -> (string=w4840:string)
                n3915 = Concatenate Strings(w4840, "\\", "Sensor File Name") -> (w4841:string)
                n3916 = local write "standard output 2"(" ") -> ()
                n3917 = String To Path(string=w4841) -> (path=w4831:path)
                n3918 = call <vilib>:"Open_Create_Replace File.vi"("advisory dialog? (display:T)"=FALSE, "function (open:0)"=T32."create or replace", "file path"=w4831) -> ("error out"=w4844:errorcluster, "refnum"=w4843:refnum<file>)  [unwired: 5 in, 2 out]
                n3919 = Set File Position(refnum=w4843, from (0:start)=w4834, error in=w4844) -> (refnum out=w4824:refnum<file>, error out=w4823:errorcluster)  [unwired: 1 in]
                n3920 = Write to Binary File(file (use dialog)=w4824, data=" ", error in=w4823, 5:FALSE ("prepend array or string size? (T)")) -> (refnum out=w4835:refnum<file>, error out=w4836:errorcluster)  [unwired: 2 in, 1 out]
                n3921 = Set File Position(offset (in bytes) (0)=w4834, refnum=w4835, error in=w4836) -> (refnum out=w4827:refnum<file>, error out=w4826:errorcluster)  [unwired: 1 in]
                n3922 = Write to Binary File(file (use dialog)=w4827, data=w4832, error in=w4826, 5:FALSE ("prepend array or string size? (T)")) -> (error out=w4830:errorcluster)  [unwired: 2 in, 2 out]
                n3923 = flat-sequence {
                  tunnel: w4831 -> [w4846]
                  tunnel: w4830 -> [_]
                  frame #0 {
                    n3924 = call <vilib>:"Read Characters From File.vi"("file path (dialog if empty)"=w4846) -> ("character string"=→"Sensor Health JSON string":string)  [unwired: 5 in, 3 out]
                  }
                }
                "SinglePoint  2" <- w4832
              }
              frame #1 {
              }
              frame #2 {
                (unwired) "\"Stored\": true" ("string")
                n3925 = call <vilib>:"System Exec.vi"("run minimized? (F)"=TRUE, "wait until completion? (T)"=TRUE, "working directory"=path "C:/LAB-IQ-NXT", "command line"="C:\\LAB-IQ-NXT\\JPostH.bat") -> ("standard error"=→"Respose From Server 2":string, "standard output"=w4851:string)  [unwired: 4 in, 2 out]
                "standard output 2" <- w4851
                n3926 = Match Pattern(string=w4851, regular expression="JSONH Check String") -> (match substring=w4849:string, offset past match=w4848:i32)  [unwired: 1 in, 2 out]
                n3927 = Equal?(x=w4849, y="JSONH Check String") -> (x = y?=→"Upload \nConfirmed 2":bool)
              }
            }
            n3928 = Divide(x=w4691, y=3600.0 ("f")) -> (x/y=w4684:dbl)
            n3929 = local read "run time"() -> (w4741:string[])
            n3930 = Round To Nearest(number=w4684) -> (nearest integer value=w4683:dbl)
            n3931 = Number To Decimal String(number=w4683) -> (decimal integer string=w4682:string)  [unwired: 1 in]
            n3932 = Index Array(array="Sensor Information", index (col) #1=0 ("disabled index (col)"), index (col) #2=1 ("index (col)"), index (col) #3=2 ("index (col)"), index (col) #4=3 ("index (col)")) -> (element #1=→"Sensor name":string[], element #2=→"model num":string[], element #3=→"run time":string[], element #4=→"state":string[])  [unwired: 4 in]
            n3933 = Insert Into Array(array=w4741, index=1, new element #1=w4682, new element #2=w4682, new element #3=w4682, new element #4=w4682, new element #5=w4682, new element #6=w4682) -> (w4706:string[])
            "run" <- w4706
            n3934 = local read "out"() -> (w4688:string[])
            n3935 = local read "Sensor Information"() -> (w4708:string[][])
            n3936 = Replace Array Subset(array=w4708, new element #1=w4706, index (col) #1=2 ("disabled index (col)"), new element #2=w4688, index (col) #2=3 ("index (col)")) -> (w4707:string[][])  [unwired: 2 in]
            n3937 = local write "Sensor Information"(w4707) -> ()
          }
        }
        n3938 = case shown="True" w4655 {
          frame False {
          }
          frame True {
            n3939 = Equal?(x="FLAG", y=0.0) -> (x = y?=w4672:bool)
            n3940 = case shown="False" w4672 {
              frame False {
                n3941 = Get Date/Time In Seconds() -> (seconds since 1Jan1904=w4678:timestamp)
                n3942 = local read "START 2"() -> (w4676:dbl)
                n3943 = To Double Precision Float(number=w4678) -> (double precision float=w4677:dbl)
                n3944 = Subtract(x=w4677, y=w4676) -> (x-y=→"SENSOR TIME  2":dbl)
              }
              frame True {
                n3945 = Get Date/Time In Seconds() -> (seconds since 1Jan1904=w4680:timestamp)
                n3946 = To Double Precision Float(number=w4680) -> (double precision float=→"START 2":dbl)
                n3947 = local write "FLAG"(100.0 ("FLAG")) -> ()
              }
            }
          }
        }
        n3948 = disable-structure shown="Disabled" {
          disable-tunnel: w4658 -> [w4667 _]
          disable-tunnel: [w4666 _] -> w4657
          frame Disabled {
            n3949 = local read "Json St Flg"() -> (w4665:bool)
            n3950 = case shown="True" w4665 {
              tunnel: w4667 -> [w4668 w4670]
              tunnel: [w4668 w4669] -> w4666
              frame False {
              }
              frame True {
                n3951 = Increment(x=w4670) -> (x+1=w4669:dbl)
                "T cycle" <- w4669
                n3952 = local write "Json St Flg"(FALSE ("Json St Flg")) -> ()
              }
            }
          }
          frame Enabled {
          }
        }
        n3953 = local read "Quit"() -> (w4652:bool)
      }
    }
    frame Enabled {
    }
  }
  n3954 = stacked-sequence {
    tunnel: [w5050] -> w38
    frame #0 {
      w5050 = FALSE ("Upload \nConfirmed")
      n3955 = local write "Upload \nConfirmed"(w5050) -> ()
      n3956 = local write "St Str"("") -> ()
    }
  }
  n3957 = disable-structure shown="Disabled" {
    disable-tunnel: w38 -> [w5051 _]
    frame Disabled {
      n3958 = case shown="True" {
        selector: _ -> [_ _]
        tunnel: w5051 -> [_ w5052]
        frame False {
        }
        frame True {
          n3959 = while {
            tunnel: [w5058] -> _
            tunnel: w5052 -> [_]
            i -> [w5058]
            stop <- w5053 stop-if-true
            n3960 = local read "Json End Flg"() -> (w5057:bool)
            n3961 = Wait (ms)(milliseconds to wait=u32 20 ("Refresh Rate (ms)")) -> ()  [unwired: 1 out]
            n3962 = local read "refresh flag"() -> (w5054:bool)
            n3963 = local read "RUN"() -> (w5055:bool)
            n3964 = And(x=w5055, y=w5054) -> (x .and. y?=w5056:bool)
            n3965 = Or(x=w5056, y=w5057) -> (x .or. y?=w5059:bool)
            "AR Led" <- w5059
            n3966 = case shown="True" w5059 {
              frame False {
              }
              frame True {
                w5076 = "\",\""
                n3967 = local read "UUID"() -> (w5074:string)
                n3968 = local write "refresh flag"(FALSE ("refresh flag")) -> ()
                n3969 = local read "time"() -> (w5063:dbl)
                n3970 = Multiply(x=w5063, y=60.0) -> (x*y=w5062:dbl)
                n3971 = Concatenate Strings("UUID\" : \"", w5074, "\"}") -> (w5077:string)
                n3972 = Number To Fractional String(number=w5062, width (-)=i16 10, precision (6)=i16 4) -> (F-format string=w5091:string)  [unwired: 1 in]
                n3973 = Concatenate Strings("{", "\"Time\":\"", w5091, w5076) -> (w5086:string)
                n3974 = stacked-sequence {
                  tunnel: w5076 -> [w5139 w5147 w5154 w5162 w5170 w5179 w5186]
                  tunnel: [w5140 _ _ _ _ _ _] -> w5090
                  tunnel: [_ w5148 _ _ _ _ _] -> w5089
                  tunnel: [_ _ w5155 _ _ _ _] -> w5088
                  tunnel: [_ _ _ w5164 _ _ _] -> w5087
                  tunnel: w5077 -> [_ _ _ _ _ _ w5197]
                  tunnel: [_ _ _ _ _ _ w5196] -> w5073
                  tunnel: [_ _ _ _ _ w5176 _] -> w5072
                  tunnel: [_ _ _ _ w5169 _ _] -> w5071
                  frame #0 {
                    n3975 = local read "NORMAL LOAD"() -> (w5138:dbl)
                    n3976 = Number To Fractional String(number=w5138, width (-)=i16 10, precision (6)=i16 4) -> (F-format string=w5141:string)  [unwired: 1 in]
                    n3977 = Concatenate Strings("NormalLoad\":\"", w5141, w5139) -> (w5140:string)
                  }
                  frame #1 {
                    n3978 = local read "Temp"() -> (w5146:dbl)
                    n3979 = Number To Fractional String(number=w5146, width (-)=i16 10, precision (6)=i16 4) -> (F-format string=w5149:string)  [unwired: 1 in]
                    n3980 = Concatenate Strings("Temperature\":\"", w5149, w5147) -> (w5148:string)
                  }
                  frame #2 {
                    n3981 = local read "cof"() -> (w5152:dbl)
                    n3982 = Number To Fractional String(number=w5152, width (-)=i16 10, precision (6)=i16 4) -> (F-format string=w5156:string)  [unwired: 1 in]
                    n3983 = Concatenate Strings("FrictionalForce\":\"", w5156, w5154) -> (w5155:string)
                  }
                  frame #3 {
                    n3984 = local read "Set Hz"() -> (w5160:dbl)
                    n3985 = Multiply(x=w5160, y=60.0) -> (x*y=w5159:dbl)
                    n3986 = Number To Fractional String(number=w5159, width (-)=i16 10, precision (6)=i16 4) -> (F-format string=w5165:string)  [unwired: 1 in]
                    n3987 = Concatenate Strings("Speed\":\"", w5165, w5162) -> (w5164:string)
                  }
                  frame #4 {
                    n3988 = local read item#-1() -> (w5168)
                    n3989 = Number To Fractional String(number=w5168, width (-)=i16 10, precision (6)=i16 4) -> (F-format string=w5172:string)  [unwired: 1 in]
                    n3990 = Concatenate Strings("LinearDeformation\":\"", w5172, w5170) -> (w5169:string)
                  }
                  frame #5 {
                    n3991 = local read "AIR TEMP"() -> (w5175:dbl)
                    n3992 = local read "Json St Flg"() -> (w5177:bool)
                    n3993 = local read "Json End Flg"() -> (w5178:bool)
                    n3994 = Number To Fractional String(number=w5175, width (-)=i16 10, precision (6)=i16 4) -> (F-format string=w5181:string)  [unwired: 1 in]
                    n3995 = Concatenate Strings("Vibration\":\"", w5181, w5179) -> (w5176:string)
                    n3996 = And(x=w5177, y=w5178) -> ()  [unwired: 1 out]
                  }
                  frame #6 {
                    n3997 = local read "Json End Flg"() -> (w5185:bool)
                    n3998 = Get Date/Time In Seconds() -> (seconds since 1Jan1904=w5193:timestamp)
                    n3999 = local read "Json St Flg"() -> (w5184:bool)
                    n4000 = To Double Precision Float(number=w5193) -> (double precision float=w5192:dbl)
                    n4001 = Subtract(x=w5192, y=2082844800.0) -> (x-y=w5190:dbl)
                    n4002 = Number To Fractional String(number=w5190, width (-)=i16 12, precision (6)=i16 0) -> (F-format string=w5187:string)  [unwired: 1 in]
                    n4003 = case shown="True" w5185 {
                      tunnel: ["" w5200] -> w5194
                      tunnel: w5187 -> [_ w5201]
                      tunnel: w5186 -> [_ w5199]
                      frame False {
                      }
                      frame True {
                        n4004 = local write "Json End Flg"(FALSE ("Json St Flg")) -> ()
                        n4005 = Concatenate Strings("End\": \"", w5201, w5199) -> (w5200:string)
                      }
                    }
                    n4006 = case shown="True" w5184 {
                      tunnel: [w5204 w5207] -> w5195
                      tunnel: w5187 -> [_ w5208]
                      tunnel: w5186 -> [_ w5205]
                      frame False {
                        n4007 = local read "St Str"() -> (w5204:string)
                      }
                      frame True {
                        n4008 = Concatenate Strings("Start\":\"", w5208, w5205) -> (w5207:string)
                        "St Str" <- w5207
                        n4009 = local write "Json St Flg"(FALSE ("Json St Flg")) -> ()
                      }
                    }
                    n4010 = Concatenate Strings(w5195, w5194, w5197) -> (w5196:string)
                  }
                }
                n4011 = local read "FILE"() -> (w5065:string)
                n4012 = Concatenate Strings("\",\"OperatorID\":\"" ("string"), "Operator ID") -> (w5068:string)
                n4013 = Concatenate Strings("\",\"DatasetTitle\":\"" ("string"), w5065) -> (w5067:string)
                n4014 = Concatenate Strings("\",\"SerialNumber\":\"" ("string"), "Serial No") -> (w5097:string)
                n4015 = Concatenate Strings("\",\"ModelNumber\":\"" ("string"), "Model No") -> (w5096:string)
                n4016 = Concatenate Strings(w5097, w5096) -> (w5079:string)
                n4017 = Concatenate Strings("{\"SecretKey\":\"", "Secret Key", w5079, w5068, w5067, "\",\"Samples\":[") -> (w5084:string)
                n4018 = Concatenate Strings(w5086, w5090, w5089, w5088, w5087, w5071, w5072, w5073) -> (w5085:string)
                n4019 = Concatenate Strings(w5084, w5085, "]}") -> (w5083:string)
                n4020 = stacked-sequence {
                  tunnel: w5083 -> [w5112 _ _]
                  tunnel: [_ _ w5129] -> _
                  frame #0 {
                    (unwired) FALSE ("convert eol (F)")
                    w5114 = enum16{"start", "end", "current"}."start" ("pos mode (0:2)")
                    n4021 = Path To String(path="Path") -> (string=w5120:string)
                    n4022 = Concatenate Strings(w5120, "\\", "Data File Name") -> (w5122:string)
                    n4023 = local write "standard output"(" ") -> ()
                    n4024 = String To Path(string=w5122) -> (path=w5111:path)
                    n4025 = call <vilib>:"Open_Create_Replace File.vi"("advisory dialog? (display:T)"=FALSE, "function (open:0)"=T32."create or replace", "file path"=w5111) -> ("error out"=w5125:errorcluster, "refnum"=w5124:refnum<file>)  [unwired: 5 in, 2 out]
                    n4026 = Set File Position(refnum=w5124, from (0:start)=w5114, error in=w5125) -> (refnum out=w5105:refnum<file>, error out=w5104:errorcluster)  [unwired: 1 in]
                    n4027 = Write to Binary File(file (use dialog)=w5105, data=" ", error in=w5104, 5:FALSE ("prepend array or string size? (T)")) -> (refnum out=w5115:refnum<file>, error out=w5116:errorcluster)  [unwired: 2 in, 1 out]
                    n4028 = Set File Position(offset (in bytes) (0)=w5114, refnum=w5115, error in=w5116) -> (refnum out=w5108:refnum<file>, error out=w5107:errorcluster)  [unwired: 1 in]
                    n4029 = Write to Binary File(file (use dialog)=w5108, data=w5112, error in=w5107, 5:FALSE ("prepend array or string size? (T)")) -> (error out=w5110:errorcluster)  [unwired: 2 in, 2 out]
                    n4030 = flat-sequence {
                      tunnel: w5111 -> [w5127]
                      tunnel: w5110 -> [_]
                      frame #0 {
                        n4031 = call <vilib>:"Read Characters From File.vi"("file path (dialog if empty)"=w5127) -> ("character string"=→"JSON string":string)  [unwired: 5 in, 3 out]
                      }
                    }
                    "SinglePoint" <- w5112
                  }
                  frame #1 {
                  }
                  frame #2 {
                    (unwired) "\"Stored\": true" ("string")
